vi "Compose Cluster - Array - Element Value.vi"() -> ()   [LabVIEW 2017, in "Composition.Tests.lvlib"]
uses:
  Composition.Tests.lvlib
  1f0bcc0f-e5b2-46f4-9ed3-af922f07b6ba.vi
  <vilib>/addons/_JKI Toolkits/Caraya/classes/Test/Test.lvclass
  <vilib>/addons/_JKI Toolkits/Caraya/classes/Assert/Assert.lvclass
panel:
  out "error out":errorcluster
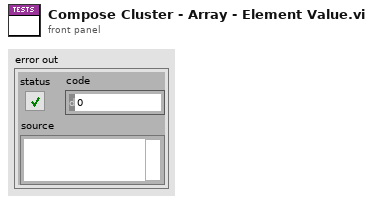
[diagram p1: front panel]
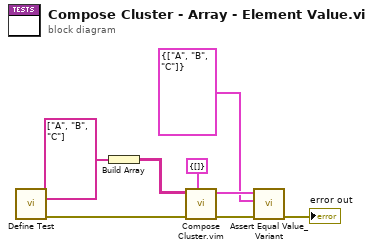
[diagram p0: block diagram]
diagram:
  n1 = call <vilib>:"Define Test.vi"() -> ("error out"=w3:errorcluster)  [unwired: 11 in]
  n2 = Build Array(string[] ["A", "B", "C"]) -> (w4:string[][])
  n3 = call "Compose Cluster.vim"("Type"=cluster{string[]} {[]}, "error in"=w3, "Elements"=w4) -> ("error out"=w6:errorcluster, "Cluster"=w2:cluster{string[]})  [unwired: 7 in]
  n4 = call <vilib>:"Assert Equal Value_Variant.vi"("error in (no error)"=w6, "Y"=cluster{string[]} {["A", "B", "C"]}, "X"=w2) -> ("error out"=→"error out":errorcluster)  [unwired: 8 in]
